vi "PH_PILS.panel.vi"(0 "object ref":refnum<vi>, 5 "error in (no error)":errorcluster) -> (19 "error out":errorcluster)   [LabVIEW 2014, in "PH_PILS.lvlib"]
doc: "By this VI a hardware switch can be monitored and switched. \n\nThe indicators \"FALSE\", \"TRUE\" and \"SWITCH STATE\" show the value of the Beckhoff-Tag: blue indicates bad tag status reference problems, darkgreen false and lightgreen true. If everything is working fine, \"FALSE\" and \"SWITCH STATE\" should show the same value, while \"TRUE\" has the opposite value. The caption of the sensors for \"FALSE\" and \"TRUE\" are taken out of the database. In case of only one or no sensor these GUI elements are not shown at all.\n\nThe oval button switches. It should be in the same state as the \"SWITCH STATE\" indicator. \n\n\"Delete Instance\" disconnects and removes the instance from the PCS.\n\n\nLicense Agreement for this software:\n\nCopyright (C)\nGesellschaft für Schwerionenforschung, GSI\nPlanckstr. 1\n64291 Darmstadt\nGermany\n\nContact: D.Beck@gsi.de \n\nThis program is free software; you can redistribute it and/or modify it under the terms of the GNU General Public License as published by the Free Software Foundation; either version 2 of the license, or (at your option) any later version.\n\nThis program is distributed in the hope that it will be useful, but WITHOUT ANYW ARRANTY; without even the implied warranty of MERCHANTABILITY or FITNESS FOR A PARTICULAR PURPOSE. See the GNU General License for more details (http://www.gnu.org).\n\nGesellschaft für Schwerionenforschung, GSI\nPlanckstr. 1, 64291 Darmstadt, Germany\nFor all questions and ideas contact: M.Richter@gsi.de, H.Brand@gsi.de or D.Beck@gsi.de.\nLast update: 18-DEC-2002"
uses:
  PH_PILS.lvlib
  PH_PILS.Submode.ctl
  PH_PILS.Operation Mode.ctl
  PH_Basics/PH_SystemInformation/PH_SystemInformation.GUI Refs.ctl
  PH_Basics/PH_Common/PH_Common.lvlib
  PH_Basics/PH_SystemInformation/PH_SystemInformation.lvlib
  PH_Basics/PH_Class/PH_Class.lvlib
  PH_Devices/PH_Beckhoff/PH_Beckhoff.lvlib
panel:
  out "PP_PA-19mm-2_DumpRoss_DE_closed_Slider":dbl(slide) scale=0.0..1.0
  out "PP_PA-19mm-1_DumpRoss_DE_closed_Slider":dbl(slide) scale=0.0..1.0
  out "PP_PA-19mm-2_DumpRoss_DE_closed":u32(colorbox)
  out "PP_PA-19mm-1_DumpRoss_DE_closed":u32(colorbox)
  out "PP_PA-19mm-2_PSU_DE_HV-on-indicator":u32(colorbox)
  out "PP_PA-19mm-1_PSU_DE_HV-on-indicator":u32(colorbox)
  out "PIL_NA_BeamdiagHVroom 2":bool caption="NA 6"
  out "PPPA_45mm_MAIN_DumpRoss_closed_Slider":dbl(slide) scale=0.0..1.0
  out "PPPA_45mm_PILC_DumpRoss_closed_Slider":dbl(slide) scale=0.0..1.0
  out "PP_PA-45mm-MAIN_DumpRoss_DE_closed":u32(colorbox)
  out "PP_PA-45mm-MAIN_PSU_DE_HV-on-indicator":u32(colorbox)
  out "PIL_DC_okPreamp":u32(colorbox)
  out "PP_Control_DC_ok":u32(colorbox)
  out "PA-19mm-Beckhoff-PU_DC_ok":u32(colorbox)
  out "PA-45mm-Beckhoff-PU_DC_ok":u32(colorbox)
  out "PIL_isOpen_T2_11":u32(colorbox)
  out "PIL_isOpen_T2_10":u32(colorbox)
  out "PIL_isOpen_T2_13":u32(colorbox)
  in  "PILo_unlock_HVDoor":bool caption="Unlock"
  in  "PILo_lock_HVDoor":bool caption="Lock"
  out "PIL_NA_BeamdiagHVroom 3":bool
  out "Mercury":u32(colorbox)=6618880 caption="23.99. 2013 08:55"
  out "PIL_Laserlab_bridged":bool caption="B"
  out "PIL_Laserbay_bridged":bool caption="B"
  in  "PILo_activate_laser_power":bool caption="Laser Suppy"
  out "PIL_Exp4_LaserEnabled":bool
  out "PIL_Exp3_LaserEnabled":bool
  out "PIL_Exp2_LaserEnabled":bool
  out "PIL_Exp1_LaserEnabled":bool
  in  "PILo_enable_AllLaser":bool
  out "PIL_disabled_laser":u32(colorbox)=16711680
  out "PPMA_Rods_b_down":u32(colorbox)
  out "PP_PA-45mm-PILC_DumpRoss_DE_closed":u32(colorbox)
  out "PIL_Shutter_Laserbay_closed":u32(colorbox)
  out "PIL_Shutter_Laserlab_closed":u32(colorbox)
  in  "PILo_activate_extEmergencies":bool
  out "PIL_Exp3_DoorOpen":u32(colorbox)
  out "PIL_Exp2_DoorOpen":u32(colorbox)
  out "PIL_Exp1_DoorOpen":u32(colorbox)
  out "MA01_O2_Lab_South_PreAlert":bool
  out "MA01_O2_Lab_North_PreAlert":bool
  out "MA-Rack4-Beckhoff-PU_DC_ok":u32(colorbox)
  out "PPMA_Rack5_DC_ok":u32(colorbox)
  out "PPMA_Rack4_DC_ok":u32(colorbox)
  out "PIL_NA_LaserLab 3":bool
  out "PA_Beckhoff-16BB_Flowbox_PA_on":bool
  out "PA_Beckhoff-16BB_Flowbox_fs_on":bool
  out "MA-Rack3-Beckhoff-PU_DC_ok":u32(colorbox)
  out "MA-Rack2-Beckhoff-PU_DC_ok":u32(colorbox)
  out "MA-Rack1-Beckhoff-PU_DC_ok":u32(colorbox)
  out "PILS_DE_earth-ok":u32(colorbox)
  out "PP_Rods_DE_watervalve-closed":bool
  out "Beamline Einschuss":u32(colorbox)
  out "PPPA_19mm_1_PSU_HV_on Head":u32(colorbox)
  out "PPPA_45mm_PSU_HV_on Head":u32(colorbox)
  out "PPPA_19mm_2_PSU_HV_on Head":u32(colorbox)
  out "PIL_shutter_fibre_closed":u32(colorbox)
  out "PIL_laserIL_deactiv 6":u32(colorbox)
  out "PIL_Lasergroup5_on 1":u32(colorbox)
  out "PIL_shutter_ns_closed":u32(colorbox)
  out "PIL_laserIL_deactiv 5":u32(colorbox)
  out "PIL_Lasergroup4_on":u32(colorbox)
  out "PIL_Lasergroup5_on 2":u32(colorbox)
  out "PIL_shutter_YLF_closed":u32(colorbox)
  out "PIL_laserIL_deactiv 4":u32(colorbox)
  out "PIL_Lasergroup2_on":u32(colorbox)
  out "PIL_shutter_Verdi_closed":u32(colorbox)
  out "PIL_laserIL_deactiv 3":u32(colorbox)
  out "PIL_Lasergroup3_on":u32(colorbox)
  out "PIL_shutter_8000B_closed":u32(colorbox)
  out "PIL_shutter_8000A_closed":u32(colorbox)
  out "PIL_laserIL_deactiv 2":u32(colorbox)
  out "PIL_shutter_9000B_closed":u32(colorbox)
  out "PIL_shutter_9000A_closed":u32(colorbox)
  out "PIL_laserIL_deactiv 1":u32(colorbox)
  out "PIL_Lasergroup1_on":u32(colorbox)
  out "Beamline Exp. 1":u32(colorbox)
  out "Beamline Exp. 2":u32(colorbox)
  out "Beamline Einschuss Exp. 1":u32(colorbox)
  out "Beamline Einschuss Exp. 2":u32(colorbox)
  out "Beamline Einschuss Exp. 3":u32(colorbox)
  out "Beamline Einschuss Exp. 4":u32(colorbox)
  out "Beamline Exp. 3":u32(colorbox)
  out "Beamline Exp. 4":u32(colorbox)
  out "Beamline Tower up":u32(colorbox)
  out "Beamline Bypass Booster":u32(colorbox)
  out "Beamline Tower/Exp":u32(colorbox)
  out "Beamline Faraday Rotator":u32(colorbox)=16711680
  out "Beamline Booster":u32(colorbox)
  out "Beamline Laserlab":u32(colorbox)
  out "Beamline MSF A":u32(colorbox)
  out "Beamline Turn MainAmp":u32(colorbox)
  out "Beamline MainAmp":u32(colorbox)
  out "PPMA_FR_PSU_HV_on Head":u32(colorbox)
  out "PPMA_PU6_PSU_HV_on Head":u32(colorbox)
  out "PPMA_PU7_PSU_HV_on Head":u32(colorbox)
  out "PPMA_PU8_PSU_HV_on Head":u32(colorbox)
  out "PPMA_PU9_PSU_HV_on Head":u32(colorbox)
  out "PPMA_PU10_PSU_HV_on Head":u32(colorbox)
  out "PPMA_PU5_PSU_HV_on Head":u32(colorbox)
  out "PPMA_PU4_PSU_HV_on Head":u32(colorbox)
  out "PPMA_PU3_PSU_HV_on Head":u32(colorbox)
  out "PPMA_PU2_PSU_HV_on Head":u32(colorbox)
  out "PPMA_PU1_PSU_HV_on Head":u32(colorbox)
  out "PPMA_Rods_a_down_Slider":dbl(slide) caption="Rods A" scale=0.0..1.0
  out "PPMA_Rods_b_down_Slider":dbl(slide) caption="Rods B" scale=0.0..1.0
  out "PPMA_Rods_a_down":u32(colorbox)
  out "PP_MA-PILC_PSU_DE_HV-on-indicator":u32(colorbox)=16860
  out "PP_MA-FR_PSU_DE_HV-on-indicator":u32(colorbox)=16860
  out "PPMA_PU10_PSU_HV_on":u32(colorbox)
  out "PPMA_PU9_PSU_HV_on":u32(colorbox)
  out "PPMA_PU8_PSU_HV_on":u32(colorbox)
  out "PPMA_PU7_PSU_HV_on":u32(colorbox)
  out "PP_MA-PU-6_PSU_DE_HV-on-indicator":u32(colorbox)
  out "PP_MA-PU-5_PSU_DE_HV-on-indicator":u32(colorbox)
  out "PP_MA-PU-4_PSU_DE_HV-on-indicator":u32(colorbox)
  out "PP_MA-PU-3_PSU_DE_HV-on-indicator":u32(colorbox)
  out "PP_MA-PU-2_PSU_DE_HV-on-indicator":u32(colorbox)
  out "PP_MA-PU-1_PSU_DE_HV-on-indicator":u32(colorbox)
  out "PILS_DE_door-locked-K2":u32(colorbox)
  out "PILS_DE_door-locked-K1":u32(colorbox)
  out "PIL_HVroom_locked":u32(colorbox)=16860
  in  "PILo_enable_exp4":bool
  out "PIL_Exp4_ShutterDisabled":u32(colorbox)
  in  "PILo_enable_exp3":bool
  out "PIL_Exp3_ShutterDisabled":u32(colorbox)
  in  "PILo_enable_exp2":bool
  out "PIL_Exp2_ShutterDisabled":u32(colorbox)
  in  "PILo_enable_exp1":bool
  out "PIL_Exp1_ShutterDisabled":u32(colorbox)
  in  "PILo_activate_MainEmergency":bool
  in  "PILo_enable_MainEmergency":bool=TRUE caption="Emergency Off"
  out "PIL_NA_Chain":u32(colorbox)
  in  "PILo_enable_Preamp":bool
  out "PIL_disabled_preamp":u32(colorbox)
  out "PIL_laserroom_ok":u32(colorbox) caption="Ack Laser Bay"
  out "PIL_HVroom_ok":u32(colorbox) caption="Ack HV"
  out "Exp":T1(ring)
  out "State Exp":u32(colorbox)
  out "Submode":T2
  out "State Submode":u32(colorbox)
  out "Operation Mode":T3
  out "State Operation Mode":u32(colorbox)
  out "PIL_Exp4_ShutterNotOpen":bool caption="Shutter not open"
  out "PIL_nhelix_on":bool caption="nhelix on"
  out "PIL_Exp4_DoorOpen":u32(colorbox)
  out "Exp. Shutter 4":dbl(slide) scale=0.0..1.0
  out "PIL_NA_Exp4":bool
  out "PIL_Exp4_ShutterNotClosed":bool caption="Shutter not closed"
  out "PIL_Exp3_ShutterNotOpen":bool caption="Shutter not open"
  out "Exp. Shutter 3":dbl(slide) scale=0.0..1.0
  out "PIL_NA_Exp3":bool
  out "PIL_Exp3_ShutterNotClosed":bool caption="Shutter not closed"
  out "PIL_Exp2_ShutterNotOpen":bool caption="Shutter not open"
  out "Exp. Shutter 2":dbl(slide) scale=0.0..1.0
  out "PIL_NA_Exp2":bool
  out "PIL_Exp2_ShutterNotClosed":bool caption="Shutter not closed"
  out "PIL_Exp1_ShutterNotOpen":bool caption="Shutter not open"
  out "Exp. Shutter 1":dbl(slide) scale=0.0..1.0
  out "PIL_NA_Exp1":bool
  out "PIL_Exp1_ShutterNotClosed":bool caption="Shutter not closed"
  out "PIL_PreAmp_keyswitch_1_002_on":u32(colorbox) caption="PP\nPA"
  out "PIL_MainAmp_keyswitch_1_002_on":u32(colorbox) caption="PP\nMA"
  out "PIL_MainAmp_keyswitch_2_005_on":u32(colorbox) caption="PP MA"
  out "PIL_DC_okA102":u32(colorbox)
  out "PPMA_Beckhoff-Dumprods_DC_ok":u32(colorbox)
  out "PIL_DC_ok11":u32(colorbox)
  out "PIL_DC_ok10":u32(colorbox)
  out "PIL_DC_ok9":u32(colorbox)
  out "PIL_DC_ok8":u32(colorbox)
  out "PIL_DC_ok7":u32(colorbox)
  out "PIL_DC_ok6":u32(colorbox)
  out "PIL_DC_ok5":u32(colorbox)
  out "PIL_DC_ok4":u32(colorbox)
  out "PIL_DC_ok3":u32(colorbox)
  out "PIL_DC_ok2":u32(colorbox)
  out "PIL_DC_ok1":u32(colorbox)
  out "PIL_NA_BeamdiagHVroom 5":bool
  out "PIL_NA_BeamdiagHVroom 4":bool
  out "PIL_enable_HVroom":bool
  in  "PILo_enable_mainamp":bool
  out "PIL_disabled_mainamp":u32(colorbox)
  out "PIL_enable_ELTroom":bool
  out "PIL_NA_LaserLab 2":bool
  out "PIL_NA_LaserLab 1":bool
  out "PIL_status_cerpass":u32(colorbox)
  out "PIL_isOpen_T1_09":u32(colorbox)
  out "PIL_isOpen_T1_10":u32(colorbox)
  out "PIL_isOpen_T1_04":u32(colorbox)
  out "PIL_isOpen_T1_05":u32(colorbox)
  out "PIL_isOpen_rollo":u32(colorbox)
  out "PIL_isOpen_T1_08":u32(colorbox)
  out "PIL_isOpen_T2_08":u32(colorbox)
  out "PIL_isOpen_T2_07":u32(colorbox)
  out "PIL_NA_PKR 1":bool
  out "PIL_NA_BeamdiagHVroom 6":bool
  out "PIL_NA_PKR 3":bool
  out "PIL_NA_PKR 2":bool
  out "PIL_NA_BeamdiagHVroom 1":bool
  out "PIL_NA_laserroom 4":bool
  out "PIL_NA_laserroom 3":bool
  out "PIL_NA_laserroom 2":bool
  out "PIL_NA_laserroom 1":bool
  out "PIL_enable_beamdiag":bool
  out "PIL_enable_laserlab":bool
  out "PIL_enable_laserroom 2":bool
  out "PIL_enable_laserroom 1":bool
  out "PIL_Exp1_MainampEnabled":bool
  out "PIL_Exp2_MainampEnabled":bool
  out "PIL_Exp3_MainampEnabled":bool
  out "PIL_Exp4_MainampEnabled":bool
  in  "Delete":bool
  # "PCS"
  # "3.40"
  # "Exp. 4 (Z6)"
  # "Experiment 1"
  # "Experiment 2"
  # "Experiment 3"
  # "LASER"
  # "Beam Diag.\nPLH 2.002"
  # "ELT  PLH 2.004"
  # "Laser Labor\nPLH 1.001"
  # "Test Labor\nPLH 2.001"
  # "HV"
  # "Stairway"
  # "Stairway"
  # "Laser Bay\nPLH 1.002"
  # "PKR\nPLH 2.007"
  # "PKR\nPLH 2.007a"
  # "HV Room\nPLH 2.005"
  # "Exp. 4 (Z6)"
  # "Exp. 3"
  # "Exp. 2"
  # "Exp. 1"
  # "EMERGENCY"
  # "PREAMP"
  # "MAINAMP"
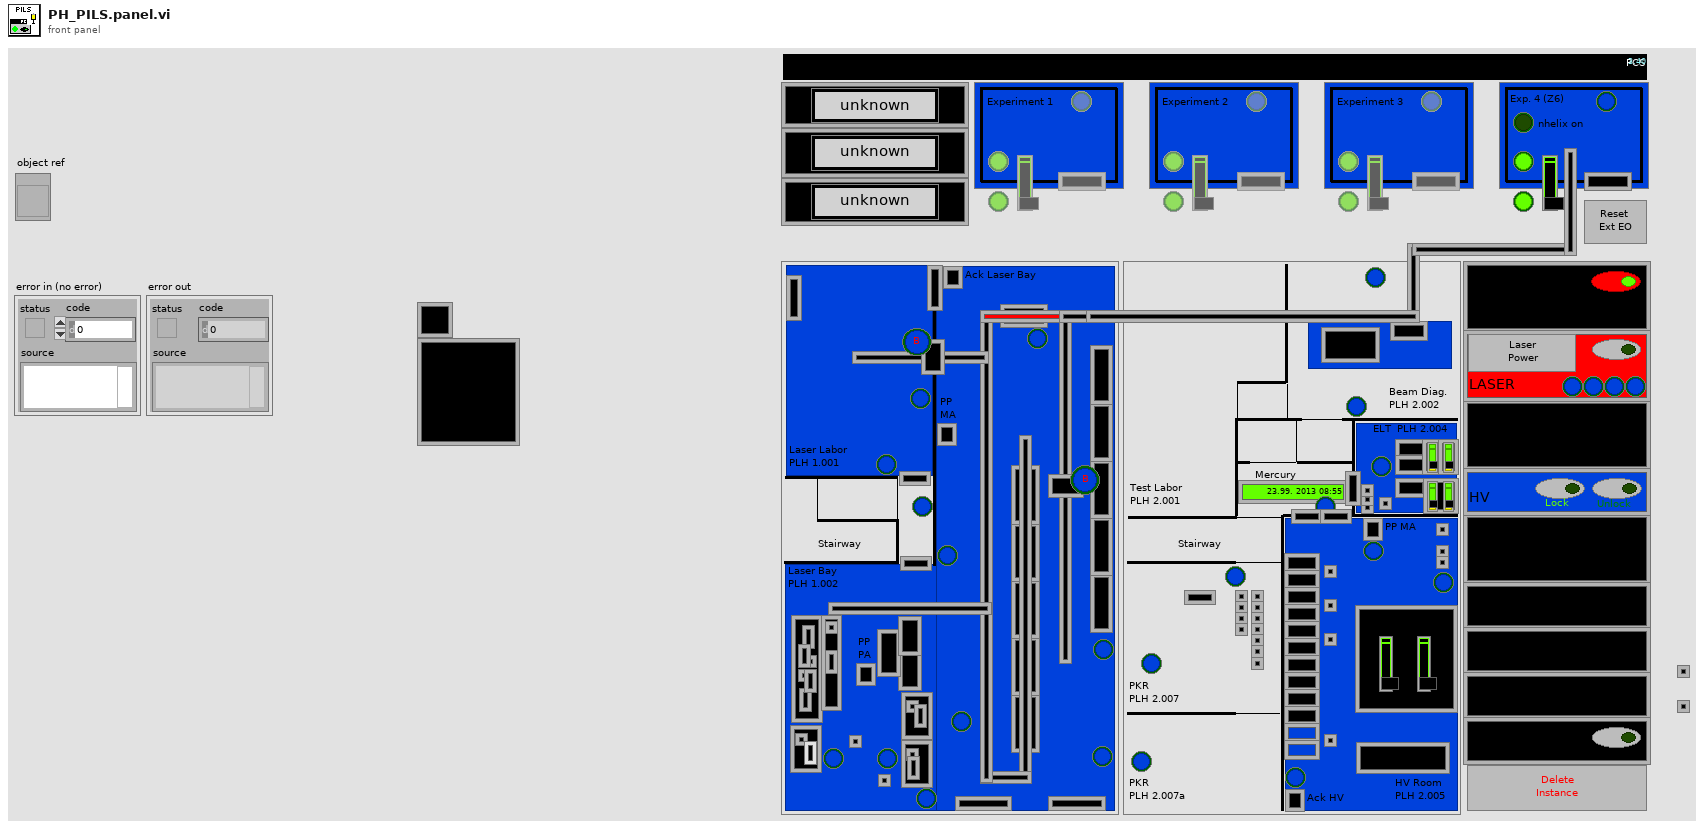
[diagram p1: front panel]
types:
  T1 = enum16{"unknown", "intern", "4 (Z6)", "3", "2", "1"}
  T2 = typedef "PH_PILS.lvlib/PH_PILS.Submode.ctl" = enum16{"unknown", "HV-Normal", "HV-Test"}
  T3 = typedef "PH_PILS.lvlib/PH_PILS.Operation Mode.ctl" = enum16{"unknown", "Service", "Labor", "Search", "Shot"}
  T4 = typedef "PH_SystemInformation.lvlib/PH_SystemInformation.GUI Refs.ctl" = cluster{"Laser":refnum<vi>, "PreAmp":refnum<vi>, "MainAmp":refnum<vi>, "Emergency Off":refnum<vi>, "Exp 1":refnum<vi>, "Exp 2":refnum<vi>, "Exp 3":refnum<vi>, "Exp 4":refnum<vi>, "Timing Mode GUI Ref":refnum<vi>}
  T5 = cluster{"GUI Ref":refnum<vi>, "Status":i32, "Head Ref":refnum<vi>, "Slider Ref":refnum<vi>}
  T6 = typedef "PH_PILS.lvlib/PH_PILS.i attribute.ctl" = cluster{"Boolean":cluster{"GUI Ref":refnum<vi>, "Status":i32}[], "GUI Refs Exp. Shutters":cluster{"1":refnum<vi>, "2":refnum<vi>, "3":refnum<vi>, "4":refnum<vi>}, "Tristate2Run GUI Refs":refnum<vi>[], "EO-Likes":cluster{"GUI Ref":refnum<vi>, "Status":i32}[], "Operation Mode":cluster{"Operation Mode":T3, "GUI":cluster{"Ref State":refnum<vi>, "Ref":refnum<vi>}, "Servicemode":cluster{"Tagname":string, "Status":i32}, "Labormode":cluster{"Tagname":string, "Status":i32}, "Searchmode":cluster{"Tagname":string, "Status":i32}, "Shotmode":cluster{"Tagname":string, "Status":i32}}, "Submode":cluster{"Submode":T2, "GUI":cluster{"Ref State":refnum<vi>, "Ref":refnum<vi>}, "Submode":cluster{"Tagname":string, "Status":i32}}, "Experiment":cluster{"Experiment":enum16{"unknown", "intern", "4 (Z6)", "3", "2", "1"}, "GUI":cluster{"Ref State":refnum<vi>, "Ref":refnum<vi>}, "intern":cluster{"Tagname":string, "Status":i32}, "Exp 4":cluster{"Tagname":string, "Status":i32}, "Exp 3":cluster{"Tagname":string, "Status":i32}, "Exp 2":cluster{"Tagname":string, "Status":i32}, "Exp 1":cluster{"Tagname":string, "Status":i32}}, "TristateNormal":cluster{"GUI Ref":refnum<vi>, "Status":i32}[], "Door Tags":cluster{"GUI Ref":refnum<vi>, "Status":i32}[], "GUIlessTags":cluster{"Name":string, "Status":i32}[], "Beamline GUI Refs":refnum<vi>[], "Special Boolean":cluster{"GUI Ref":refnum<vi>, "Status":i32}[], "Laserpower":cluster{"GUI Ref":refnum<vi>, "Status":i32}[], "Shutter":cluster{"GUI Ref":refnum<vi>, "Status":i32}[], "Tristate EO Like":cluster{"GUI Ref":refnum<vi>, "Status":i32}[], "PP":cluster{"GUI Ref":refnum<vi>, "Status":i32, "Head Ref":refnum<vi>, "Slider Ref":refnum<vi>}[], "Switch Knobs":cluster{"GUI Ref":refnum<vi>, "Status":i32}[], "Latch Knob GUI Refs":refnum<vi>[], "FailureCounter":i32, "Enabled Status":cluster{"Laser":i32, "PreAmp":i32, "MainAmp":i32}, "Mercury":refnum<vi>, "Instance Rods":string, "Logfile":path, "Beckhoff-Instance Internal":string, "Beckhoff-Instance External":string, "Enabling Rights":cluster{"Name":string, "Password":string, "PA?":bool, "MA?":bool, "Exp?":bool}[]}
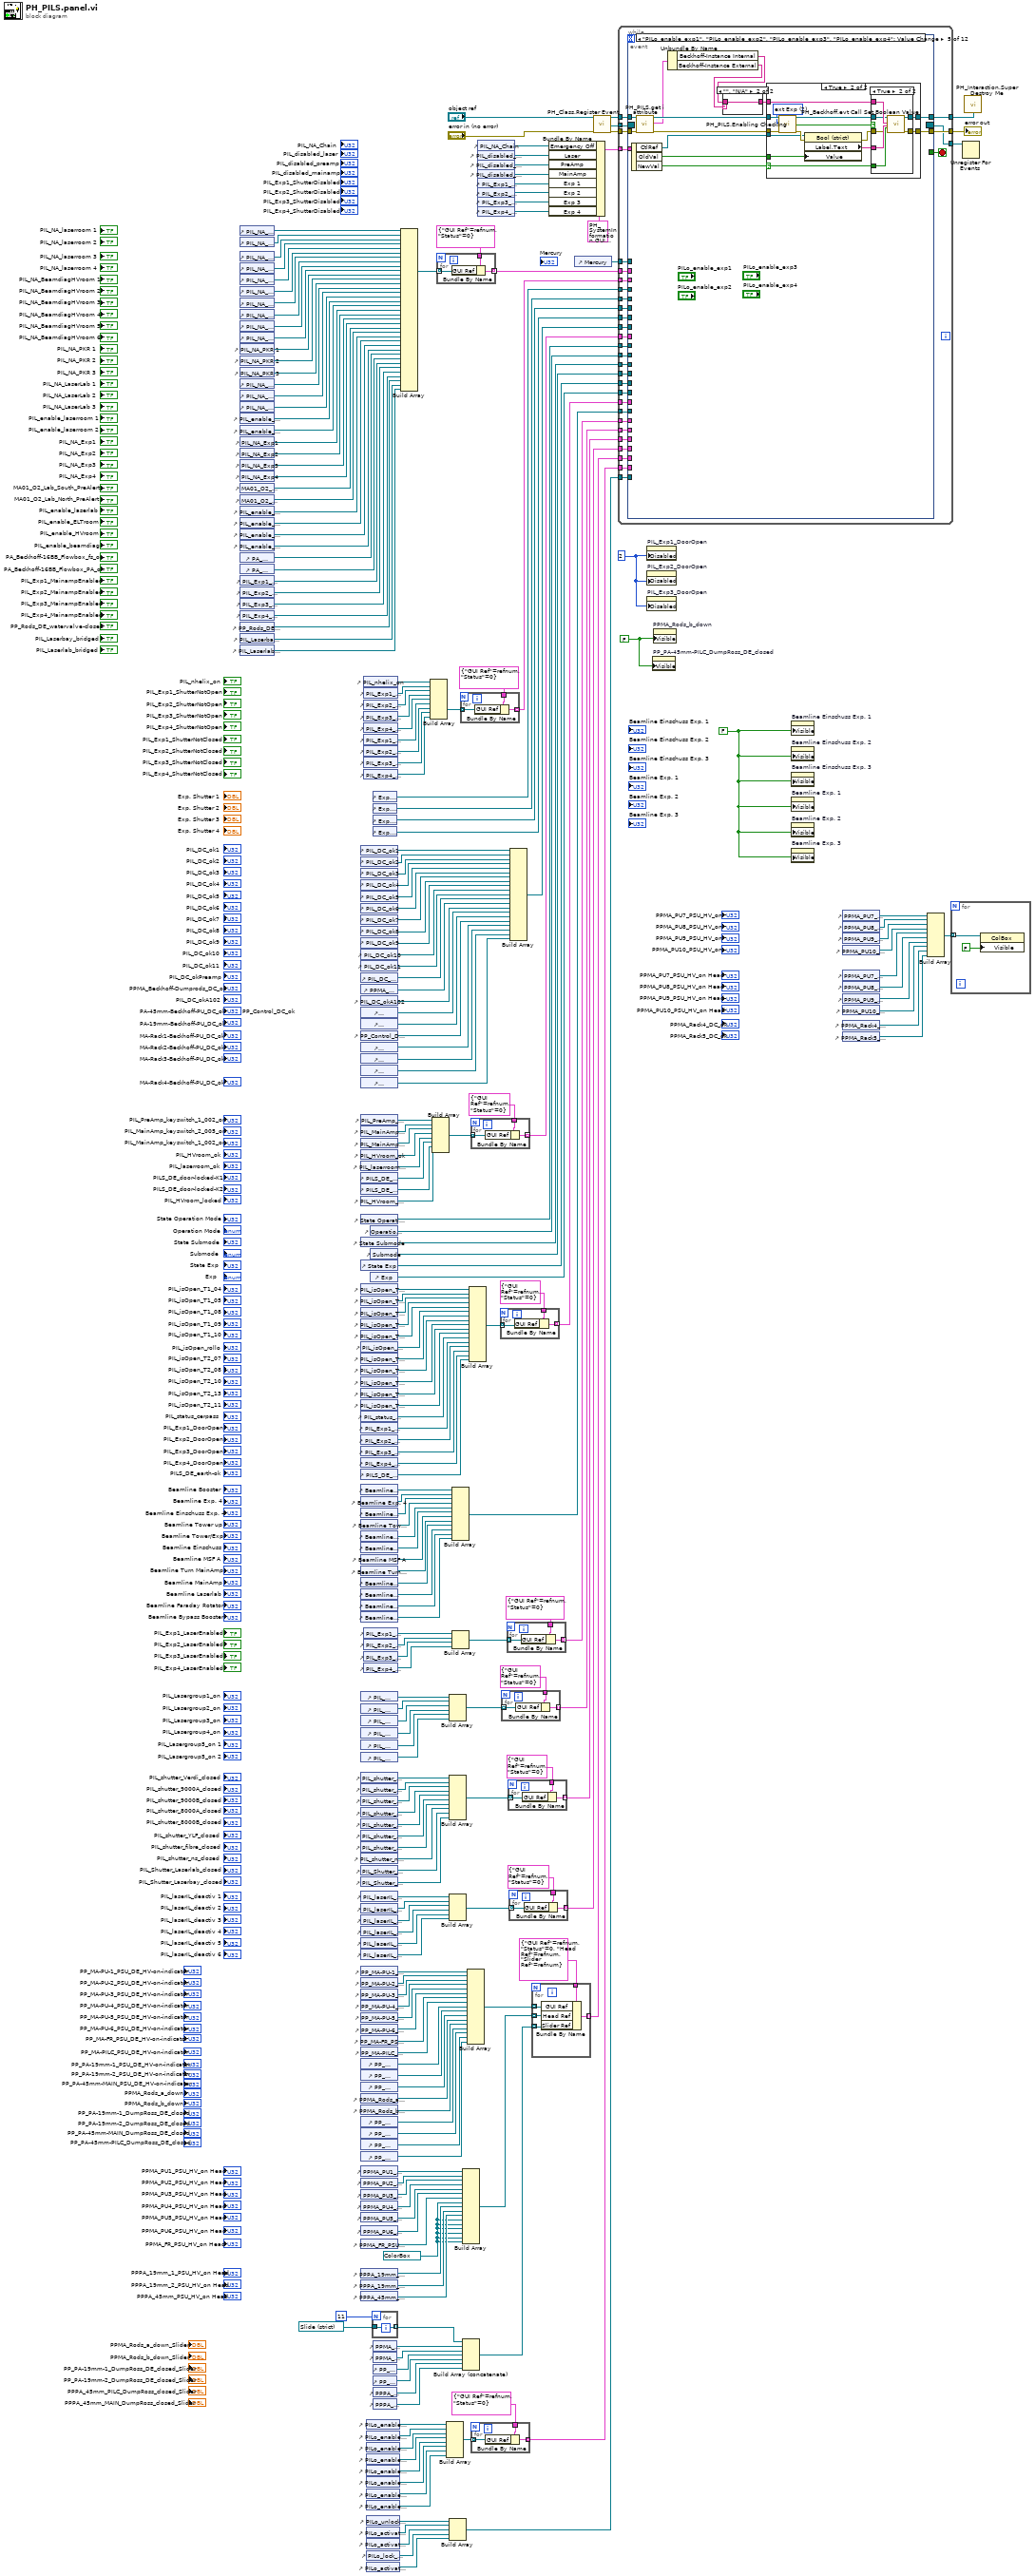
[diagram p0: block diagram]
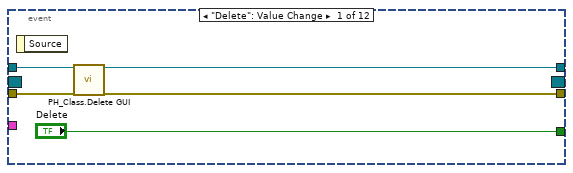
[diagram p2: hidden frame]
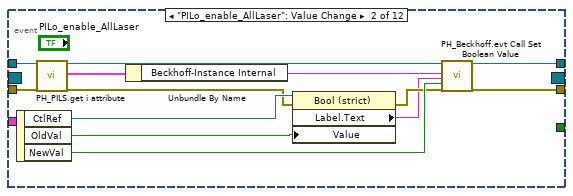
[diagram p3: hidden frame]
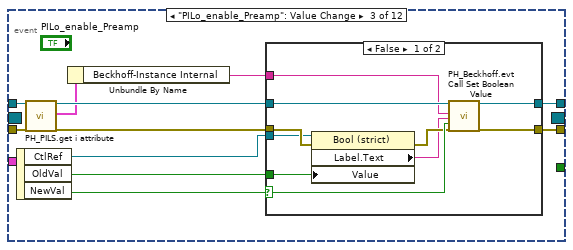
[diagram p4: hidden frame]
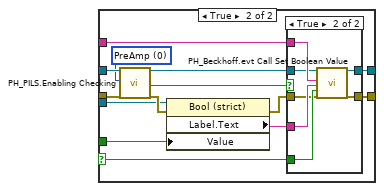
[diagram p5: hidden frame]
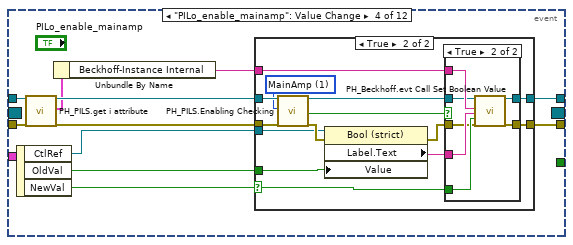
[diagram p7: hidden frame]
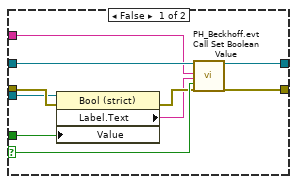
[diagram p8: hidden frame]
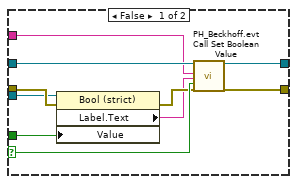
[diagram p11: hidden frame]
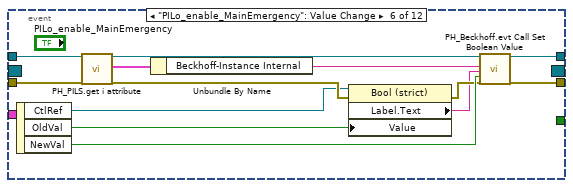
[diagram p13: hidden frame]
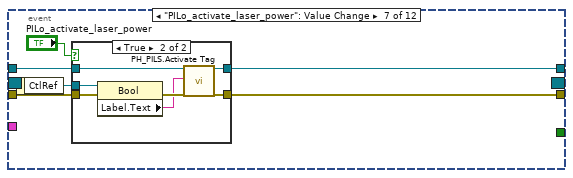
[diagram p14: hidden frame]
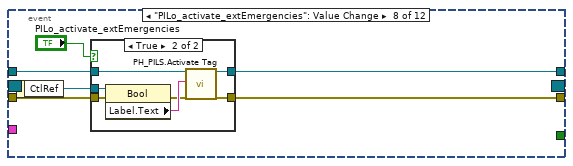
[diagram p16: hidden frame]
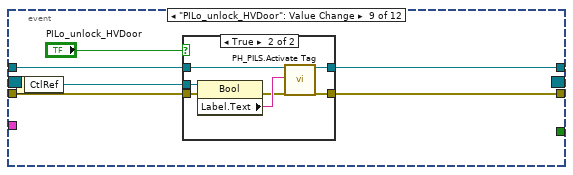
[diagram p18: hidden frame]
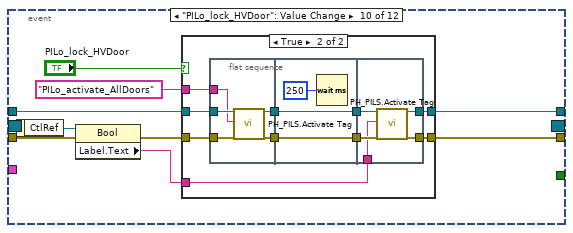
[diagram p20: hidden frame]
diagram:
  w77 = u8 2 ("Disabled")
  w90 = refnum<vi> refnum ("PPPA_45mm_PSU_HV_on Head")
  w98 = FALSE ("Visible")
  w171 = FALSE ("Visible")
  n1 = control-ref of="PIL_NA_laserroom 1"() -> (w257:refnum<vi>)
  n2 = control-ref of="PIL_NA_laserroom 2"() -> (w256:refnum<vi>)
  n3 = control-ref of="PIL_NA_laserroom 3"() -> (w255:refnum<vi>)
  n4 = control-ref of="PIL_NA_laserroom 4"() -> (w254:refnum<vi>)
  n5 = control-ref of="PIL_NA_BeamdiagHVroom 1"() -> (w253:refnum<vi>)
  n6 = control-ref of="PIL_NA_BeamdiagHVroom 2"() -> (w252:refnum<vi>)
  n7 = control-ref of="PIL_NA_BeamdiagHVroom 3"() -> (w251:refnum<vi>)
  n8 = control-ref of="PIL_NA_BeamdiagHVroom 4"() -> (w250:refnum<vi>)
  n9 = control-ref of="PIL_NA_BeamdiagHVroom 5"() -> (w249:refnum<vi>)
  n10 = control-ref of="PIL_NA_BeamdiagHVroom 6"() -> (w248:refnum<vi>)
  n11 = control-ref of="PIL_NA_PKR 1"() -> (w247:refnum<vi>)
  n12 = control-ref of="PIL_NA_PKR 2"() -> (w246:refnum<vi>)
  n13 = control-ref of="PIL_NA_PKR 3"() -> (w245:refnum<vi>)
  n14 = control-ref of="PIL_NA_LaserLab 1"() -> (w244:refnum<vi>)
  n15 = control-ref of="PIL_NA_LaserLab 2"() -> (w243:refnum<vi>)
  n16 = control-ref of="PIL_NA_LaserLab 3"() -> (w242:refnum<vi>)
  n17 = control-ref of="PIL_enable_laserroom 1"() -> (w241:refnum<vi>)
  n18 = control-ref of="PIL_enable_laserroom 2"() -> (w240:refnum<vi>)
  n19 = control-ref of="PIL_NA_Exp1"() -> (w239:refnum<vi>)
  n20 = control-ref of="PIL_NA_Exp2"() -> (w238:refnum<vi>)
  n21 = control-ref of="PIL_NA_Exp3"() -> (w237:refnum<vi>)
  n22 = control-ref of="PIL_NA_Exp4"() -> (w236:refnum<vi>)
  n23 = control-ref of="MA01_O2_Lab_South_PreAlert"() -> (w235:refnum<vi>)
  n24 = control-ref of="MA01_O2_Lab_North_PreAlert"() -> (w234:refnum<vi>)
  n25 = control-ref of="PIL_enable_laserlab"() -> (w233:refnum<vi>)
  n26 = control-ref of="PIL_enable_ELTroom"() -> (w232:refnum<vi>)
  n27 = control-ref of="PIL_enable_HVroom"() -> (w231:refnum<vi>)
  n28 = control-ref of="PIL_enable_beamdiag"() -> (w230:refnum<vi>)
  n29 = control-ref of="PA_Beckhoff-16BB_Flowbox_fs_on"() -> (w229:refnum<vi>)
  n30 = control-ref of="PA_Beckhoff-16BB_Flowbox_PA_on"() -> (w228:refnum<vi>)
  n31 = control-ref of="PIL_Exp1_MainampEnabled"() -> (w227:refnum<vi>)
  n32 = control-ref of="PIL_Exp2_MainampEnabled"() -> (w226:refnum<vi>)
  n33 = control-ref of="PIL_Exp3_MainampEnabled"() -> (w225:refnum<vi>)
  n34 = control-ref of="PIL_Exp4_MainampEnabled"() -> (w224:refnum<vi>)
  n35 = control-ref of="PP_Rods_DE_watervalve-closed"() -> (w223:refnum<vi>)
  n36 = control-ref of="PIL_Laserbay_bridged"() -> (w47:refnum<vi>)
  n37 = control-ref of="PIL_Laserlab_bridged"() -> (w46:refnum<vi>)
  n38 = control-ref of="PIL_DC_ok1"() -> (w211:refnum<vi>)
  n39 = control-ref of="PIL_DC_ok2"() -> (w210:refnum<vi>)
  n40 = control-ref of="PIL_DC_ok3"() -> (w209:refnum<vi>)
  n41 = control-ref of="PIL_DC_ok4"() -> (w208:refnum<vi>)
  n42 = control-ref of="PIL_DC_ok5"() -> (w207:refnum<vi>)
  n43 = control-ref of="PIL_DC_ok6"() -> (w206:refnum<vi>)
  n44 = control-ref of="PIL_DC_ok7"() -> (w205:refnum<vi>)
  n45 = control-ref of="PIL_DC_ok8"() -> (w204:refnum<vi>)
  n46 = control-ref of="PIL_DC_ok9"() -> (w203:refnum<vi>)
  n47 = control-ref of="PIL_DC_ok10"() -> (w202:refnum<vi>)
  n48 = control-ref of="PIL_DC_ok11"() -> (w201:refnum<vi>)
  n49 = control-ref of="PIL_DC_okPreamp"() -> (w200:refnum<vi>)
  n50 = control-ref of="PPMA_Beckhoff-Dumprods_DC_ok"() -> (w199:refnum<vi>)
  n51 = control-ref of="PIL_DC_okA102"() -> (w198:refnum<vi>)
  n52 = control-ref of="PA-45mm-Beckhoff-PU_DC_ok"() -> (w197:refnum<vi>)
  n53 = control-ref of="PA-19mm-Beckhoff-PU_DC_ok"() -> (w196:refnum<vi>)
  n54 = control-ref of="PP_Control_DC_ok"() -> (w195:refnum<vi>)
  n55 = control-ref of="MA-Rack1-Beckhoff-PU_DC_ok"() -> (w60:refnum<vi>)
  n56 = control-ref of="MA-Rack2-Beckhoff-PU_DC_ok"() -> (w59:refnum<vi>)
  n57 = control-ref of="MA-Rack3-Beckhoff-PU_DC_ok"() -> (w58:refnum<vi>)
  n58 = control-ref of="MA-Rack4-Beckhoff-PU_DC_ok"() -> (w57:refnum<vi>)
  n59 = control-ref of="PIL_PreAmp_keyswitch_1_002_on"() -> (w194:refnum<vi>)
  n60 = control-ref of="PIL_MainAmp_keyswitch_2_005_on"() -> (w193:refnum<vi>)
  n61 = control-ref of="PIL_MainAmp_keyswitch_1_002_on"() -> (w192:refnum<vi>)
  n62 = control-ref of="PIL_HVroom_ok"() -> (w191:refnum<vi>)
  n63 = control-ref of="PIL_laserroom_ok"() -> (w190:refnum<vi>)
  n64 = control-ref of="PILS_DE_door-locked-K1"() -> (w189:refnum<vi>)
  n65 = control-ref of="PILS_DE_door-locked-K2"() -> (w188:refnum<vi>)
  n66 = control-ref of="PIL_HVroom_locked"() -> (w130:refnum<vi>)
  n67 = control-ref of="State Operation Mode"() -> (w15:refnum<vi>)
  n68 = control-ref of="State Submode"() -> (w13:refnum<vi>)
  n69 = control-ref of="State Exp"() -> (w11:refnum<vi>)
  n70 = control-ref of="PIL_isOpen_T1_04"() -> (w183:refnum<vi>)
  n71 = control-ref of="PIL_isOpen_T1_05"() -> (w182:refnum<vi>)
  n72 = control-ref of="PIL_isOpen_T1_08"() -> (w181:refnum<vi>)
  n73 = control-ref of="PIL_isOpen_T1_09"() -> (w180:refnum<vi>)
  n74 = control-ref of="PIL_isOpen_T1_10"() -> (w144:refnum<vi>)
  n75 = control-ref of="PIL_isOpen_rollo"() -> (w179:refnum<vi>)
  n76 = control-ref of="PIL_isOpen_T2_07"() -> (w178:refnum<vi>)
  n77 = control-ref of="PIL_isOpen_T2_08"() -> (w177:refnum<vi>)
  n78 = control-ref of="PIL_isOpen_T2_10"() -> (w176:refnum<vi>)
  n79 = control-ref of="PIL_isOpen_T2_13"() -> (w175:refnum<vi>)
  n80 = control-ref of="PIL_isOpen_T2_11"() -> (w174:refnum<vi>)
  n81 = control-ref of="PIL_status_cerpass"() -> (w173:refnum<vi>)
  n82 = control-ref of="PIL_Exp1_DoorOpen"() -> (w121:refnum<vi>)
  n83 = control-ref of="PIL_Exp2_DoorOpen"() -> (w120:refnum<vi>)
  n84 = control-ref of="PIL_Exp3_DoorOpen"() -> (w119:refnum<vi>)
  n85 = control-ref of="PIL_Exp4_DoorOpen"() -> (w118:refnum<vi>)
  n86 = control-ref of="PILS_DE_earth-ok"() -> (w78:refnum<vi>)
  n87 = control-ref of="Beamline Booster"() -> (w170:refnum<vi>)
  n88 = control-ref of="Beamline Exp. 4"() -> (w169:refnum<vi>)
  n89 = control-ref of="Beamline Einschuss Exp. 4"() -> (w168:refnum<vi>)
  n90 = control-ref of="Beamline Tower up"() -> (w167:refnum<vi>)
  n91 = control-ref of="Beamline Tower/Exp"() -> (w166:refnum<vi>)
  n92 = control-ref of="Beamline Einschuss"() -> (w165:refnum<vi>)
  n93 = control-ref of="Beamline MSF A"() -> (w164:refnum<vi>)
  n94 = control-ref of="Beamline Turn MainAmp"() -> (w163:refnum<vi>)
  n95 = control-ref of="Beamline MainAmp"() -> (w162:refnum<vi>)
  n96 = control-ref of="Beamline Laserlab"() -> (w161:refnum<vi>)
  n97 = control-ref of="Beamline Faraday Rotator"() -> (w160:refnum<vi>)
  n98 = control-ref of="Beamline Bypass Booster"() -> (w159:refnum<vi>)
  n99 = control-ref of="PIL_Lasergroup1_on"() -> (w152:refnum<vi>)
  n100 = control-ref of="PIL_Lasergroup2_on"() -> (w151:refnum<vi>)
  n101 = control-ref of="PIL_Lasergroup3_on"() -> (w150:refnum<vi>)
  n102 = control-ref of="PIL_Lasergroup4_on"() -> (w149:refnum<vi>)
  n103 = control-ref of="PIL_Lasergroup5_on 1"() -> (w148:refnum<vi>)
  n104 = control-ref of="PIL_Lasergroup5_on 2"() -> (w147:refnum<vi>)
  n105 = control-ref of="PIL_shutter_Verdi_closed"() -> (w143:refnum<vi>)
  n106 = control-ref of="PIL_shutter_9000A_closed"() -> (w142:refnum<vi>)
  n107 = control-ref of="PIL_shutter_9000B_closed"() -> (w141:refnum<vi>)
  n108 = control-ref of="PIL_shutter_8000A_closed"() -> (w140:refnum<vi>)
  n109 = control-ref of="PIL_shutter_8000B_closed"() -> (w139:refnum<vi>)
  n110 = control-ref of="PIL_shutter_YLF_closed"() -> (w138:refnum<vi>)
  n111 = control-ref of="PIL_shutter_fibre_closed"() -> (w137:refnum<vi>)
  n112 = control-ref of="PIL_shutter_ns_closed"() -> (w136:refnum<vi>)
  n113 = control-ref of="PIL_Shutter_Laserlab_closed"() -> (w135:refnum<vi>)
  n114 = control-ref of="PIL_Shutter_Laserbay_closed"() -> (w134:refnum<vi>)
  n115 = control-ref of="PIL_laserIL_deactiv 1"() -> (w129:refnum<vi>)
  n116 = control-ref of="PIL_laserIL_deactiv 2"() -> (w128:refnum<vi>)
  n117 = control-ref of="PIL_laserIL_deactiv 3"() -> (w127:refnum<vi>)
  n118 = control-ref of="PIL_laserIL_deactiv 4"() -> (w126:refnum<vi>)
  n119 = control-ref of="PIL_laserIL_deactiv 5"() -> (w124:refnum<vi>)
  n120 = control-ref of="PIL_laserIL_deactiv 6"() -> (w125:refnum<vi>)
  n121 = control-ref of="PP_MA-PU-1_PSU_DE_HV-on-indicator"() -> (w117:refnum<vi>)
  n122 = control-ref of="PP_MA-PU-2_PSU_DE_HV-on-indicator"() -> (w116:refnum<vi>)
  n123 = control-ref of="PP_MA-PU-3_PSU_DE_HV-on-indicator"() -> (w115:refnum<vi>)
  n124 = control-ref of="PP_MA-PU-4_PSU_DE_HV-on-indicator"() -> (w114:refnum<vi>)
  n125 = control-ref of="PP_MA-PU-5_PSU_DE_HV-on-indicator"() -> (w113:refnum<vi>)
  n126 = control-ref of="PP_MA-PU-6_PSU_DE_HV-on-indicator"() -> (w34:refnum<vi>)
  n127 = control-ref of="PP_MA-FR_PSU_DE_HV-on-indicator"() -> (w112:refnum<vi>)
  n128 = control-ref of="PP_MA-PILC_PSU_DE_HV-on-indicator"() -> (w33:refnum<vi>)
  n129 = control-ref of="PP_PA-19mm-1_PSU_DE_HV-on-indicator"() -> (w111:refnum<vi>)
  n130 = control-ref of="PP_PA-19mm-2_PSU_DE_HV-on-indicator"() -> (w110:refnum<vi>)
  n131 = control-ref of="PP_PA-45mm-MAIN_PSU_DE_HV-on-indicator"() -> (w109:refnum<vi>)
  n132 = control-ref of="PPMA_Rods_a_down"() -> (w97:refnum<vi>)
  n133 = control-ref of="PPMA_Rods_b_down"() -> (w96:refnum<vi>)
  n134 = control-ref of="PP_PA-19mm-1_DumpRoss_DE_closed"() -> (w95:refnum<vi>)
  n135 = control-ref of="PP_PA-19mm-2_DumpRoss_DE_closed"() -> (w94:refnum<vi>)
  n136 = control-ref of="PP_PA-45mm-MAIN_DumpRoss_DE_closed"() -> (w93:refnum<vi>)
  n137 = control-ref of="PP_PA-45mm-PILC_DumpRoss_DE_closed"() -> (w92:refnum<vi>)
  n138 = control-ref of="PPMA_PU1_PSU_HV_on Head"() -> (w107:refnum<vi>)
  n139 = control-ref of="PPMA_PU2_PSU_HV_on Head"() -> (w106:refnum<vi>)
  n140 = control-ref of="PPMA_PU3_PSU_HV_on Head"() -> (w105:refnum<vi>)
  n141 = control-ref of="PPMA_PU4_PSU_HV_on Head"() -> (w104:refnum<vi>)
  n142 = control-ref of="PPMA_PU5_PSU_HV_on Head"() -> (w103:refnum<vi>)
  n143 = control-ref of="PPMA_PU6_PSU_HV_on Head"() -> (w32:refnum<vi>)
  n144 = control-ref of="PPMA_FR_PSU_HV_on Head"() -> (w102:refnum<vi>)
  n145 = control-ref of="PPPA_19mm_1_PSU_HV_on Head"() -> (w101:refnum<vi>)
  n146 = control-ref of="PPPA_19mm_2_PSU_HV_on Head"() -> (w100:refnum<vi>)
  n147 = control-ref of="PPPA_45mm_PSU_HV_on Head"() -> (w99:refnum<vi>)
  n148 = control-ref of="PIL_nhelix_on"() -> (w222:refnum<vi>)
  n149 = control-ref of="PIL_Exp1_ShutterNotOpen"() -> (w221:refnum<vi>)
  n150 = control-ref of="PIL_Exp2_ShutterNotOpen"() -> (w220:refnum<vi>)
  n151 = control-ref of="PIL_Exp3_ShutterNotOpen"() -> (w219:refnum<vi>)
  n152 = control-ref of="PIL_Exp4_ShutterNotOpen"() -> (w218:refnum<vi>)
  n153 = control-ref of="PIL_Exp1_ShutterNotClosed"() -> (w217:refnum<vi>)
  n154 = control-ref of="PIL_Exp2_ShutterNotClosed"() -> (w216:refnum<vi>)
  n155 = control-ref of="PIL_Exp3_ShutterNotClosed"() -> (w215:refnum<vi>)
  n156 = control-ref of="PIL_Exp4_ShutterNotClosed"() -> (w214:refnum<vi>)
  n157 = control-ref of="PIL_Exp1_LaserEnabled"() -> (w158:refnum<vi>)
  n158 = control-ref of="PIL_Exp2_LaserEnabled"() -> (w157:refnum<vi>)
  n159 = control-ref of="PIL_Exp3_LaserEnabled"() -> (w156:refnum<vi>)
  n160 = control-ref of="PIL_Exp4_LaserEnabled"() -> (w155:refnum<vi>)
  n161 = control-ref of="PILo_enable_MainEmergency"() -> (w76:refnum<vi>)
  n162 = control-ref of="PILo_enable_AllLaser"() -> (w75:refnum<vi>)
  n163 = control-ref of="PILo_enable_Preamp"() -> (w74:refnum<vi>)
  n164 = control-ref of="PILo_enable_mainamp"() -> (w73:refnum<vi>)
  n165 = control-ref of="PILo_enable_exp1"() -> (w72:refnum<vi>)
  n166 = control-ref of="PILo_enable_exp2"() -> (w71:refnum<vi>)
  n167 = control-ref of="PILo_enable_exp3"() -> (w67:refnum<vi>)
  n168 = control-ref of="PILo_enable_exp4"() -> (w70:refnum<vi>)
  n169 = control-ref of="PILo_unlock_HVDoor"() -> (w66:refnum<vi>)
  n170 = control-ref of="PILo_activate_MainEmergency"() -> (w65:refnum<vi>)
  n171 = control-ref of="PILo_activate_extEmergencies"() -> (w64:refnum<vi>)
  n172 = control-ref of="PILo_lock_HVDoor"() -> (w63:refnum<vi>)
  n173 = control-ref of="PILo_activate_laser_power"() -> (w62:refnum<vi>)
  n174 = control-ref of="Operation Mode"() -> (w14:refnum<vi>)
  n175 = control-ref of="Submode"() -> (w12:refnum<vi>)
  n176 = control-ref of="Exp"() -> (w10:refnum<vi>)
  n177 = for {
    N: 11 -> [_]
    tunnel: [w259] -> w80 mode=indexing
    tunnel: refnum<vi> refnum ("PPPA_19mm_1_DumpRoss_closed_Slider") -> [w259]
  }
  n178 = control-ref of="Exp. Shutter 1"() -> (w21:refnum<vi>)
  n179 = control-ref of="Exp. Shutter 2"() -> (w20:refnum<vi>)
  n180 = control-ref of="Exp. Shutter 3"() -> (w19:refnum<vi>)
  n181 = control-ref of="Exp. Shutter 4"() -> (w18:refnum<vi>)
  n182 = control-ref of="PPMA_Rods_a_down_Slider"() -> (w84:refnum<vi>)
  n183 = control-ref of="PPMA_Rods_b_down_Slider"() -> (w83:refnum<vi>)
  n184 = control-ref of="PP_PA-19mm-1_DumpRoss_DE_closed_Slider"() -> (w89:refnum<vi>)
  n185 = control-ref of="PP_PA-19mm-2_DumpRoss_DE_closed_Slider"() -> (w88:refnum<vi>)
  n186 = control-ref of="PPPA_45mm_PILC_DumpRoss_closed_Slider"() -> (w87:refnum<vi>)
  n187 = control-ref of="PPPA_45mm_MAIN_DumpRoss_closed_Slider"() -> (w86:refnum<vi>)
  n188 = Build Array(w257, w256, w255, w254, w253, w252, w251, w250, w249, w248, w247, w246, w245, w244, w243, w242, w241, w240, w239, w238, w237, w236, w235, w234, w233, w232, w231, w230, w229, w228, w227, w226, w225, w224, w223, w47, w46) -> (w186:refnum<vi>[])
  n189 = Build Array(w222, w221, w220, w219, w218, w217, w216, w215, w214) -> (w213:refnum<vi>[])
  n190 = Build Array(w194, w193, w192, w191, w190, w189, w188, w130) -> (w185:refnum<vi>[])
  n191 = for {
    tunnel: cluster{"GUI Ref":refnum<vi>, "Status":i32} {"GUI Ref"=refnum, "Status"=0} ("Cluster") -> [w262]
    tunnel: w186 -> [w260] mode=indexing
    tunnel: [w261] -> w23 mode=indexing
    n192 = Bundle By Name(cluster=w262, "GUI Ref"=w260) -> (w261:cluster{"GUI Ref":refnum<vi>, "Status":i32})
  }
  n193 = Build Array(w76, w75, w74, w73, w72, w71, w67, w70) -> (w68:refnum<vi>[])
  n194 = Build Array(w66, w65, w64, w63, w62) -> (w1:refnum<vi>[])
  n195 = Build Array(w152, w151, w150, w149, w148, w147) -> (w145:refnum<vi>[])
  n196 = Build Array(w143, w142, w141, w140, w139, w138, w137, w136, w135, w134) -> (w132:refnum<vi>[])
  n197 = Build Array(w129, w128, w127, w126, w124, w125) -> (w122:refnum<vi>[])
  n198 = Build Array(w170, w169, w168, w167, w166, w165, w164, w163, w162, w161, w160, w159) -> (w8:refnum<vi>[])
  n199 = Build Array(w158, w157, w156, w155) -> (w153:refnum<vi>[])
  n200 = for {
    tunnel: cluster{"GUI Ref":refnum<vi>, "Status":i32} {"GUI Ref"=refnum, "Status"=0} ("Cluster") -> [w265]
    tunnel: w213 -> [w263] mode=indexing
    tunnel: [w264] -> w22 mode=indexing
    n201 = Bundle By Name(cluster=w265, "GUI Ref"=w263) -> (w264:cluster{"GUI Ref":refnum<vi>, "Status":i32})
  }
  n202 = Build Array(w107, w106, w105, w104, w103, w32, w102, w90, w101, w100, w99, w90, w90, w90, w90, w90, w90) -> (w91:refnum<vi>[])
  n203 = Build Array (concatenate)(w80, w84, w83, w89, w88, w87, w86) -> (w79:refnum<vi>[])
  n204 = Build Array(w117, w116, w115, w114, w113, w34, w112, w33, w111, w110, w109, w97, w96, w95, w94, w93, w92) -> (w108:refnum<vi>[])
  n205 = Build Array(w183, w182, w181, w180, w144, w179, w178, w177, w176, w175, w174, w173, w121, w120, w119, w118, w78) -> (w172:refnum<vi>[])
  n206 = for {
    tunnel: cluster{"GUI Ref":refnum<vi>, "Status":i32} {"GUI Ref"=refnum, "Status"=0} ("element") -> [w268]
    tunnel: w185 -> [w266] mode=indexing
    tunnel: [w267] -> w16 mode=indexing
    n207 = Bundle By Name(cluster=w268, "GUI Ref"=w266) -> (w267:cluster{"GUI Ref":refnum<vi>, "Status":i32})
  }
  n208 = for {
    tunnel: cluster{"GUI Ref":refnum<vi>, "Status":i32} {"GUI Ref"=refnum, "Status"=0} ("Cluster") -> [w271]
    tunnel: [w270] -> w2 mode=indexing
    tunnel: w68 -> [w269] mode=indexing
    n209 = Bundle By Name(cluster=w271, "GUI Ref"=w269) -> (w270:cluster{"GUI Ref":refnum<vi>, "Status":i32})
  }
  n210 = control-ref of="PIL_NA_Chain"() -> (w55:refnum<vi>)
  n211 = control-ref of="PIL_disabled_laser"() -> (w54:refnum<vi>)
  n212 = control-ref of="PIL_disabled_preamp"() -> (w53:refnum<vi>)
  n213 = control-ref of="PIL_disabled_mainamp"() -> (w52:refnum<vi>)
  n214 = control-ref of="PIL_Exp1_ShutterDisabled"() -> (w51:refnum<vi>)
  n215 = control-ref of="PIL_Exp2_ShutterDisabled"() -> (w50:refnum<vi>)
  n216 = control-ref of="PIL_Exp3_ShutterDisabled"() -> (w49:refnum<vi>)
  n217 = control-ref of="PIL_Exp4_ShutterDisabled"() -> (w48:refnum<vi>)
  n218 = for {
    tunnel: cluster{"GUI Ref":refnum<vi>, "Status":i32} {"GUI Ref"=refnum, "Status"=0} ("element") -> [w274]
    tunnel: w172 -> [w272] mode=indexing
    tunnel: [w273] -> w9 mode=indexing
    n219 = Bundle By Name(cluster=w274, "GUI Ref"=w272) -> (w273:cluster{"GUI Ref":refnum<vi>, "Status":i32})
  }
  n220 = for {
    tunnel: cluster{"GUI Ref":refnum<vi>, "Status":i32} {"GUI Ref"=refnum, "Status"=0} ("element") -> [w277]
    tunnel: w145 -> [w275] mode=indexing
    tunnel: [w276] -> w6 mode=indexing
    n221 = Bundle By Name(cluster=w277, "GUI Ref"=w275) -> (w276:cluster{"GUI Ref":refnum<vi>, "Status":i32})
  }
  n222 = for {
    tunnel: cluster{"GUI Ref":refnum<vi>, "Status":i32} {"GUI Ref"=refnum, "Status"=0} ("Cluster") -> [w280]
    tunnel: w153 -> [w278] mode=indexing
    tunnel: [w279] -> w7 mode=indexing
    n223 = Bundle By Name(cluster=w280, "GUI Ref"=w278) -> (w279:cluster{"GUI Ref":refnum<vi>, "Status":i32})
  }
  n224 = for {
    tunnel: cluster{"GUI Ref":refnum<vi>, "Status":i32} {"GUI Ref"=refnum, "Status"=0} ("element") -> [w283]
    tunnel: w132 -> [w281] mode=indexing
    tunnel: [w282] -> w5 mode=indexing
    n225 = Bundle By Name(cluster=w283, "GUI Ref"=w281) -> (w282:cluster{"GUI Ref":refnum<vi>, "Status":i32})
  }
  n226 = for {
    tunnel: cluster{"GUI Ref":refnum<vi>, "Status":i32} {"GUI Ref"=refnum, "Status"=0} ("element") -> [w286]
    tunnel: w122 -> [w284] mode=indexing
    tunnel: [w285] -> w4 mode=indexing
    n227 = Bundle By Name(cluster=w286, "GUI Ref"=w284) -> (w285:cluster{"GUI Ref":refnum<vi>, "Status":i32})
  }
  n228 = Build Array(w211, w210, w209, w208, w207, w206, w205, w204, w203, w202, w201, w200, w199, w198, w197, w196, w195, w60, w59, w58, w57) -> (w17:refnum<vi>[])
  n229 = for {
    tunnel: T5 {"GUI Ref"=refnum, "Status"=0, "Head Ref"=refnum, "Slider Ref"=refnum} ("Cluster") -> [w291]
    tunnel: w108 -> [w289] mode=indexing
    tunnel: [w290] -> w3 mode=indexing
    tunnel: w91 -> [w288] mode=indexing
    tunnel: w79 -> [w287] mode=indexing
    n230 = Bundle By Name(cluster=w291, "GUI Ref"=w289, "Head Ref"=w288, "Slider Ref"=w287) -> (w290:T5)
  }
  n231 = Bundle By Name(cluster=T4 {"Laser"=refnum, "PreAmp"=refnum, "MainAmp"=refnum, "Emergency Off"=refnum, "Exp 1"=refnum, "Exp 2"=refnum, "Exp 3"=refnum, "Exp 4"=refnum, "Timing Mode GUI Ref"=refnum} ("GUI Refs"), "Emergency Off"=w55, "Laser"=w54, "PreAmp"=w53, "MainAmp"=w52, "Exp 1"=w51, "Exp 2"=w50, "Exp 3"=w49, "Exp 4"=w48) -> (w27:T4)
  n232 = control-ref of="Mercury"() -> (w24:refnum<vi>)
  n233 = call "PH_Class.Register Event.vi"("i ref in"="object ref", "error in (no error)"="error in (no error)") -> ("i ref out"=w30:refnum<vi>, "Event Registration Refnum"=w29:refnum<event-registration>, "error out"=w31:errorcluster)  [unwired: 15 in]
  n234 = while {
    tunnel: w30 -> [w320]
    tunnel: [w319] -> w61
    tunnel: w31 -> [w322]
    tunnel: [w321] -> w258
    tunnel: w29 -> [w318]
    tunnel: [w317] -> w28
    tunnel: w27 -> [w316]
    tunnel: w24 -> [w315]
    tunnel: w23 -> [w314]
    tunnel: w22 -> [w313]
    tunnel: w21 -> [w312]
    tunnel: w20 -> [w311]
    tunnel: w19 -> [w310]
    tunnel: w18 -> [w309]
    tunnel: w17 -> [w308]
    tunnel: w16 -> [w307]
    tunnel: w15 -> [w306]
    tunnel: w14 -> [w305]
    tunnel: w13 -> [w304]
    tunnel: w12 -> [w303]
    tunnel: w11 -> [w302]
    tunnel: w10 -> [w301]
    tunnel: w9 -> [w300]
    tunnel: w8 -> [w299]
    tunnel: w7 -> [w298]
    tunnel: w6 -> [w297]
    tunnel: w5 -> [w296]
    tunnel: w4 -> [w295]
    tunnel: w3 -> [w294]
    tunnel: w2 -> [w293]
    tunnel: w1 -> [w292]
    stop <- w323 stop-if-true
    n235 = event shown="[4] \"PILo_enable_exp1\", \"PILo_enable_exp2\", \"PILo_enable_exp3\", \"PILo_enable_exp4\": Value Change" {
      selector: w318 -> [_ _ _ _ _ _ _ _ _ _ _ _]
      dyn-events: [_ _ _ _ _ _ _ _ _ _ _ _] -> w317
      timeout: _ -> [_ _ _ _ _ _ _ _ _ _ _ _]
      tunnel: ["Delete" _ _ _ _ _ _ _ _ _ _ _] -> w323
      tunnel: w320 -> [w327 w341 w352 w396 w442 w490 w493 w508 w523 w541 w577 w636]
      tunnel: w322 -> [w326 w340 w351 w395 w441 w489 w492 w507 w522 w540 w576 w635]
      tunnel: [w325 w337 w348 w392 w438 w486 w495 w510 w525 w543 w579 w607] -> w321
      tunnel: [w324 w338 w349 w393 w439 w487 w496 w511 w526 w544 w580 w605] -> w319
      tunnel: w316 -> [_ _ _ _ _ _ _ _ _ _ _ w632]
      tunnel: w315 -> [_ _ _ _ _ _ _ _ _ _ _ w631]
      tunnel: w314 -> [_ _ _ _ _ _ _ _ _ _ _ w630]
      tunnel: w313 -> [_ _ _ _ _ _ _ _ _ _ _ w629]
      tunnel: w312 -> [_ _ _ _ _ _ _ _ _ _ _ w628]
      tunnel: w311 -> [_ _ _ _ _ _ _ _ _ _ _ w627]
      tunnel: w310 -> [_ _ _ _ _ _ _ _ _ _ _ w626]
      tunnel: w309 -> [_ _ _ _ _ _ _ _ _ _ _ w625]
      tunnel: w308 -> [_ _ _ _ _ _ _ _ _ _ _ w624]
      tunnel: w307 -> [_ _ _ _ _ _ _ _ _ _ _ w623]
      tunnel: w306 -> [_ _ _ _ _ _ _ _ _ _ _ w622]
      tunnel: w305 -> [_ _ _ _ _ _ _ _ _ _ _ w621]
      tunnel: w304 -> [_ _ _ _ _ _ _ _ _ _ _ w620]
      tunnel: w303 -> [_ _ _ _ _ _ _ _ _ _ _ w619]
      tunnel: w302 -> [_ _ _ _ _ _ _ _ _ _ _ w618]
      tunnel: w301 -> [_ _ _ _ _ _ _ _ _ _ _ w617]
      tunnel: w300 -> [_ _ _ _ _ _ _ _ _ _ _ w616]
      tunnel: w299 -> [_ _ _ _ _ _ _ _ _ _ _ w615]
      tunnel: w298 -> [_ _ _ _ _ _ _ _ _ _ _ w614]
      tunnel: w297 -> [_ _ _ _ _ _ _ _ _ _ _ w613]
      tunnel: w296 -> [_ _ _ _ _ _ _ _ _ _ _ w612]
      tunnel: w295 -> [_ _ _ _ _ _ _ _ _ _ _ w611]
      tunnel: w294 -> [_ _ _ _ _ _ _ _ _ _ _ w610]
      tunnel: w293 -> [_ _ _ _ _ _ _ _ _ _ _ w609]
      tunnel: w292 -> [_ _ _ _ _ _ _ _ _ _ _ w608]
      event "Delete": Value Change {
        n236 = event-data() -> ()  [unwired: 1 in, 1 out]
        n237 = call "PH_Class.Delete GUI.vi"("VI in"=w327, "error in (no error)"=w326) -> ("VI out"=w324:refnum<vi>, "error out"=w325:errorcluster)  [unwired: 16 in]
      }
      event "PILo_enable_AllLaser": Value Change {
        n238 = event-data() -> ("CtlRef"=w335:refnum<vi>, "OldVal"=w331:bool, "NewVal"=w336:bool)  [unwired: 1 in]
        n239 = call "PH_PILS.get i attribute.vi"("i ref in"=w341, "error in (no error)"=w340) -> ("i ref out"=w339:refnum<vi>, "i attribute"=w330:T6, "error out"=w334:errorcluster)  [unwired: 15 in]
        n240 = Unbundle By Name(w330) -> ("Beckhoff-Instance Internal"=w329:string)
        n241 = property class="Bool (strict)"(reference=w335, error in=w334, "Value"=w331) -> (error out=w333:errorcluster, "Label.Text"=w332:string)  [unwired: 1 out]
        n242 = call "PH_Beckhoff.evt Call Set Boolean Value.vi"("i ref in"=w339, "Beckhoff Instance"=w329, "Tagname to set"=w332, "Value"=w336, "error in"=w333) -> ("i ref out"=w338:refnum<vi>, "error out"=w337:errorcluster)  [unwired: 13 in]
      }
      event "PILo_enable_Preamp": Value Change {
        n243 = event-data() -> ("CtlRef"=w344:refnum<vi>, "OldVal"=w345:bool, "NewVal"=w347:bool)  [unwired: 1 in]
        n244 = call "PH_PILS.get i attribute.vi"("i ref in"=w352, "error in (no error)"=w351) -> ("i ref out"=w350:refnum<vi>, "i attribute"=w343:T6, "error out"=w346:errorcluster)  [unwired: 15 in]
        n245 = Unbundle By Name(w343) -> ("Beckhoff-Instance Internal"=w342:string)
        n246 = case shown="False" w347 {
          selector: w347 -> [w359 w374]
          tunnel: w350 -> [w362 w373]
          tunnel: [w361 w376] -> w349
          tunnel: [w360 w375] -> w348
          tunnel: w346 -> [w358 w369]
          tunnel: w342 -> [w353 w363]
          tunnel: w345 -> [w355 w365]
          tunnel: w344 -> [w356 w364]
          frame False {
            n247 = property class="Bool (strict)"(reference=w356, error in=w358, "Value"=w355) -> (error out=w357:errorcluster, "Label.Text"=w354:string)  [unwired: 1 out]
            n248 = call "PH_Beckhoff.evt Call Set Boolean Value.vi"("i ref in"=w362, "Beckhoff Instance"=w353, "Tagname to set"=w354, "Value"=w359, "error in"=w357) -> ("i ref out"=w361:refnum<vi>, "error out"=w360:errorcluster)  [unwired: 13 in]
          }
          frame True {
            w371 = u16 0 items=["PreAmp", "MainAmp", "ext Exp"] ("System to enable")
            n249 = call "PH_PILS.Enabling Checking.vi"("i ref in"=w373, "System to enable"=w371, "error in"=w369) -> ("i ref out"=w372:refnum<vi>, "Enabling allowed"=w370:bool, "error out"=w368:errorcluster)  [unwired: 14 in]
            n250 = property class="Bool (strict)"(reference=w364, error in=w368, "Value"=w365) -> (error out=w367:errorcluster, "Label.Text"=w366:string)  [unwired: 1 out]
            n251 = case shown="True" w370 {
              tunnel: [w378 w385] -> w376
              tunnel: [w377 w384] -> w375
              tunnel: w363 -> [_ w383]
              tunnel: w366 -> [_ w382]
              tunnel: w374 -> [_ w381]
              tunnel: w367 -> [w377 w380]
              tunnel: w372 -> [w378 w379]
              frame False {
              }
              frame True {
                n252 = call "PH_Beckhoff.evt Call Set Boolean Value.vi"("i ref in"=w379, "Beckhoff Instance"=w383, "Tagname to set"=w382, "Value"=w381, "error in"=w380) -> ("i ref out"=w385:refnum<vi>, "error out"=w384:errorcluster)  [unwired: 13 in]
              }
            }
          }
        }
      }
      event "PILo_enable_mainamp": Value Change {
        n253 = event-data() -> ("CtlRef"=w388:refnum<vi>, "OldVal"=w389:bool, "NewVal"=w391:bool)  [unwired: 1 in]
        n254 = call "PH_PILS.get i attribute.vi"("i ref in"=w396, "error in (no error)"=w395) -> ("i ref out"=w394:refnum<vi>, "i attribute"=w387:T6, "error out"=w390:errorcluster)  [unwired: 15 in]
        n255 = Unbundle By Name(w387) -> ("Beckhoff-Instance Internal"=w386:string)
        n256 = case shown="True" w391 {
          selector: w391 -> [w403 w418]
          tunnel: w394 -> [w406 w417]
          tunnel: [w405 w420] -> w393
          tunnel: [w404 w419] -> w392
          tunnel: w390 -> [w402 w413]
          tunnel: w386 -> [w397 w407]
          tunnel: w389 -> [w399 w409]
          tunnel: w388 -> [w400 w408]
          frame False {
            n257 = property class="Bool (strict)"(reference=w400, error in=w402, "Value"=w399) -> (error out=w401:errorcluster, "Label.Text"=w398:string)  [unwired: 1 out]
            n258 = call "PH_Beckhoff.evt Call Set Boolean Value.vi"("i ref in"=w406, "Beckhoff Instance"=w397, "Tagname to set"=w398, "Value"=w403, "error in"=w401) -> ("i ref out"=w405:refnum<vi>, "error out"=w404:errorcluster)  [unwired: 13 in]
          }
          frame True {
            w415 = u16 1 items=["PreAmp", "MainAmp", "ext Exp"] ("System to enable")
            n259 = call "PH_PILS.Enabling Checking.vi"("i ref in"=w417, "System to enable"=w415, "error in"=w413) -> ("i ref out"=w416:refnum<vi>, "Enabling allowed"=w414:bool, "error out"=w412:errorcluster)  [unwired: 14 in]
            n260 = property class="Bool (strict)"(reference=w408, error in=w412, "Value"=w409) -> (error out=w411:errorcluster, "Label.Text"=w410:string)  [unwired: 1 out]
            n261 = case shown="True" w414 {
              tunnel: [w422 w429] -> w420
              tunnel: [w421 w428] -> w419
              tunnel: w407 -> [_ w427]
              tunnel: w410 -> [_ w426]
              tunnel: w418 -> [_ w425]
              tunnel: w411 -> [w421 w424]
              tunnel: w416 -> [w422 w423]
              frame False {
              }
              frame True {
                n262 = call "PH_Beckhoff.evt Call Set Boolean Value.vi"("i ref in"=w423, "Beckhoff Instance"=w427, "Tagname to set"=w426, "Value"=w425, "error in"=w424) -> ("i ref out"=w429:refnum<vi>, "error out"=w428:errorcluster)  [unwired: 13 in]
              }
            }
          }
        }
      }
      event "PILo_enable_exp1", "PILo_enable_exp2", "PILo_enable_exp3", "PILo_enable_exp4": Value Change {
        n263 = event-data() -> ("CtlRef"=w434:refnum<vi>, "OldVal"=w435:bool, "NewVal"=w437:bool)  [unwired: 1 in]
        n264 = call "PH_PILS.get i attribute.vi"("i ref in"=w442, "error in (no error)"=w441) -> ("i ref out"=w440:refnum<vi>, "i attribute"=w433:T6, "error out"=w436:errorcluster)  [unwired: 15 in]
        n265 = Unbundle By Name(w433) -> ("Beckhoff-Instance Internal"=w431:string, "Beckhoff-Instance External"=w430:string)
        n266 = case shown="\"\", \"N/A\"" w430 {
          selector: w430 -> [w443 _]
          tunnel: [w443 w444] -> w432
          tunnel: w431 -> [_ w444]
          frame Default {
          }
          frame "", "N/A" {
          }
        }
        n267 = case shown="True" w437 {
          selector: w437 -> [w451 w466]
          tunnel: w440 -> [w454 w465]
          tunnel: [w453 w468] -> w439
          tunnel: [w452 w467] -> w438
          tunnel: w436 -> [w450 w461]
          tunnel: w432 -> [w445 w455]
          tunnel: w435 -> [w447 w457]
          tunnel: w434 -> [w448 w456]
          frame False {
            n268 = property class="Bool (strict)"(reference=w448, error in=w450, "Value"=w447) -> (error out=w449:errorcluster, "Label.Text"=w446:string)  [unwired: 1 out]
            n269 = call "PH_Beckhoff.evt Call Set Boolean Value.vi"("i ref in"=w454, "Beckhoff Instance"=w445, "Tagname to set"=w446, "Value"=w451, "error in"=w449) -> ("i ref out"=w453:refnum<vi>, "error out"=w452:errorcluster)  [unwired: 13 in]
          }
          frame True {
            w463 = u16 2 items=["PreAmp", "MainAmp", "ext Exp"] ("System to enable")
            n270 = call "PH_PILS.Enabling Checking.vi"("i ref in"=w465, "System to enable"=w463, "error in"=w461) -> ("i ref out"=w464:refnum<vi>, "Enabling allowed"=w462:bool, "error out"=w460:errorcluster)  [unwired: 14 in]
            n271 = property class="Bool (strict)"(reference=w456, error in=w460, "Value"=w457) -> (error out=w459:errorcluster, "Label.Text"=w458:string)  [unwired: 1 out]
            n272 = case shown="True" w462 {
              tunnel: [w470 w477] -> w468
              tunnel: [w469 w476] -> w467
              tunnel: w455 -> [_ w475]
              tunnel: w458 -> [_ w474]
              tunnel: w466 -> [_ w473]
              tunnel: w459 -> [w469 w472]
              tunnel: w464 -> [w470 w471]
              frame False {
              }
              frame True {
                n273 = call "PH_Beckhoff.evt Call Set Boolean Value.vi"("i ref in"=w471, "Beckhoff Instance"=w475, "Tagname to set"=w474, "Value"=w473, "error in"=w472) -> ("i ref out"=w477:refnum<vi>, "error out"=w476:errorcluster)  [unwired: 13 in]
              }
            }
          }
        }
      }
      event "PILo_enable_MainEmergency": Value Change {
        n274 = event-data() -> ("CtlRef"=w482:refnum<vi>, "OldVal"=w483:bool, "NewVal"=w485:bool)  [unwired: 1 in]
        n275 = call "PH_PILS.get i attribute.vi"("i ref in"=w490, "error in (no error)"=w489) -> ("i ref out"=w488:refnum<vi>, "i attribute"=w479:T6, "error out"=w484:errorcluster)  [unwired: 15 in]
        n276 = Unbundle By Name(w479) -> ("Beckhoff-Instance Internal"=w478:string)
        n277 = property class="Bool (strict)"(reference=w482, error in=w484, "Value"=w483) -> (error out=w481:errorcluster, "Label.Text"=w480:string)  [unwired: 1 out]
        n278 = call "PH_Beckhoff.evt Call Set Boolean Value.vi"("i ref in"=w488, "Beckhoff Instance"=w478, "Tagname to set"=w480, "Value"=w485, "error in"=w481) -> ("i ref out"=w487:refnum<vi>, "error out"=w486:errorcluster)  [unwired: 13 in]
      }
      event "PILo_activate_laser_power": Value Change {
        n279 = event-data() -> ("CtlRef"=w494:refnum<vi>)  [unwired: 1 in]
        n280 = case shown="True" "PILo_activate_laser_power" {
          tunnel: [w498 w505] -> w496
          tunnel: [w497 w504] -> w495
          tunnel: w494 -> [_ w502]
          tunnel: w493 -> [w498 w500]
          tunnel: w492 -> [w497 w499]
          frame False {
          }
          frame True {
            n281 = property class="Bool"(reference=w502, error in=w499) -> (error out=w503:errorcluster, "Label.Text"=w501:string)  [unwired: 1 out]
            n282 = call "PH_PILS.Activate Tag.vi"("i ref in"=w500, "Tag Name"=w501, "error in (no error)"=w503) -> ("i ref out"=w505:refnum<vi>, "error out"=w504:errorcluster)  [unwired: 15 in]
          }
        }
      }
      event "PILo_activate_extEmergencies": Value Change {
        n283 = event-data() -> ("CtlRef"=w509:refnum<vi>)  [unwired: 1 in]
        n284 = case shown="True" "PILo_activate_extEmergencies" {
          tunnel: [w513 w520] -> w511
          tunnel: [w512 w519] -> w510
          tunnel: w509 -> [_ w518]
          tunnel: w508 -> [w513 w515]
          tunnel: w507 -> [w512 w516]
          frame False {
          }
          frame True {
            n285 = property class="Bool"(reference=w518, error in=w516) -> (error out=w514:errorcluster, "Label.Text"=w517:string)  [unwired: 1 out]
            n286 = call "PH_PILS.Activate Tag.vi"("i ref in"=w515, "Tag Name"=w517, "error in (no error)"=w514) -> ("i ref out"=w520:refnum<vi>, "error out"=w519:errorcluster)  [unwired: 15 in]
          }
        }
      }
      event "PILo_unlock_HVDoor": Value Change {
        n287 = event-data() -> ("CtlRef"=w524:refnum<vi>)  [unwired: 1 in]
        n288 = case shown="True" "PILo_unlock_HVDoor" {
          tunnel: [w528 w535] -> w526
          tunnel: [w527 w534] -> w525
          tunnel: w524 -> [_ w533]
          tunnel: w523 -> [w528 w531]
          tunnel: w522 -> [w527 w530]
          frame False {
          }
          frame True {
            n289 = property class="Bool"(reference=w533, error in=w530) -> (error out=w529:errorcluster, "Label.Text"=w532:string)  [unwired: 1 out]
            n290 = call "PH_PILS.Activate Tag.vi"("i ref in"=w531, "Tag Name"=w532, "error in (no error)"=w529) -> ("i ref out"=w535:refnum<vi>, "error out"=w534:errorcluster)  [unwired: 15 in]
          }
        }
      }
      event "PILo_lock_HVDoor": Value Change {
        n291 = event-data() -> ("CtlRef"=w542:refnum<vi>)  [unwired: 1 in]
        n292 = property class="Bool"(reference=w542, error in=w540) -> (error out=w539:errorcluster, "Label.Text"=w536:string)  [unwired: 1 out]
        n293 = case shown="True" "PILo_lock_HVDoor" {
          tunnel: [w546 w556] -> w544
          tunnel: [w545 w555] -> w543
          tunnel: w541 -> [w546 w548]
          tunnel: w539 -> [w545 w547]
          tunnel: "PILo_activate_AllDoors" -> [_ w554]
          tunnel: w536 -> [_ w549]
          frame False {
          }
          frame True {
            n294 = flat-sequence {
              tunnel: w548 -> [w559]
              tunnel: w547 -> [w558]
              tunnel: w554 -> [w557]
              tunnel: [w561] -> w553
              tunnel: [w560] -> w552
              tunnel: w553 -> [w564]
              tunnel: w552 -> [w563]
              tunnel: [w564] -> w551
              tunnel: [w563] -> w550
              tunnel: [w566] -> w555
              tunnel: [w567] -> w556
              tunnel: w551 -> [w569]
              tunnel: w550 -> [w568]
              tunnel: w549 -> [w565]
              frame #0 {
                n295 = call "PH_PILS.Activate Tag.vi"("i ref in"=w559, "Tag Name"=w557, "error in (no error)"=w558) -> ("i ref out"=w561:refnum<vi>, "error out"=w560:errorcluster)  [unwired: 15 in]
              }
              frame #1 {
                n296 = Wait (ms)(milliseconds to wait=u32 250) -> ()  [unwired: 1 out]
              }
              frame #2 {
                n297 = call "PH_PILS.Activate Tag.vi"("i ref in"=w569, "Tag Name"=w565, "error in (no error)"=w568) -> ("i ref out"=w567:refnum<vi>, "error out"=w566:errorcluster)  [unwired: 15 in]
              }
            }
          }
        }
      }
      event "PILo_activate_MainEmergency": Value Change {
        n298 = event-data() -> ("CtlRef"=w578:refnum<vi>)  [unwired: 1 in]
        n299 = property class="Bool"(reference=w578, error in=w576) -> (error out=w575:errorcluster, "Label.Text"=w573:string)  [unwired: 1 out]
        n300 = Build Array("PILo_activate_subEmergencies", "PILo_activate_extEmergencies", w573) -> (w572:string[])
        n301 = case shown="True" "PILo_activate_MainEmergency" {
          tunnel: [w582 w592] -> w580
          tunnel: [w581 w591] -> w579
          tunnel: w577 -> [w582 w596]
          tunnel: w575 -> [w581 w599]
          tunnel: w572 -> [_ w598]
          frame False {
          }
          frame True {
            n302 = call "PH_PILS.get i attribute.vi"("i ref in"=w596, "error in (no error)"=w599) -> ("i ref out"=w595:refnum<vi>, "i attribute"=w584:T6, "error out"=w597:errorcluster)  [unwired: 15 in]
            n303 = Unbundle By Name(w584) -> ("Logfile"=w583:path)
            n304 = Open/Create/Replace File(file path (use dialog)=w583) -> (refnum out=w588:refnum<file>, error out=w587:errorcluster)  [unwired: 5 in, 1 out]
            n305 = Set File Position(refnum=w588, from (0:start)=enum16{"start", "end", "current"}."end", error in=w587) -> (refnum out=w586:refnum<file>, error out=w585:errorcluster)  [unwired: 1 in]
            n306 = call "PH_PILS.Dialog EO.vi"() -> ("EO Comment"=w589:string)
            n307 = for {
              tunnel: w598 -> [w600] mode=indexing
              shift-right: [w604] -> w592
              shift-left: w595 -> [w602]
              shift-right: [w603] -> w591
              shift-left: w597 -> [w601]
              n308 = call "PH_PILS.Activate Tag.vi"("i ref in"=w602, "Tag Name"=w600, "error in (no error)"=w601) -> ("i ref out"=w604:refnum<vi>, "error out"=w603:errorcluster)  [unwired: 15 in]
            }
            n309 = Write to Text File(file (use dialog)=w586, text=w589, error in=w585) -> (refnum out=w594:refnum<file>, error out=w593:errorcluster)  [unwired: 1 in, 1 out]
            n310 = Close File(refnum=w594, error in=w593) -> ()  [unwired: 2 out]
          }
        }
      }
      event User Event {
        n311 = event-data() -> ("Class"=w634:string)  [unwired: 1 in]
        n312 = case shown="\"PH_PILS\"" w634 {
          selector: w634 -> [w637 _]
          tunnel: w636 -> [w642 w670]
          tunnel: [w641 w644] -> w606
          tunnel: w635 -> [w640 w669]
          tunnel: [w639 w643] -> w633
          tunnel: w632 -> [w638 _]
          tunnel: w631 -> [_ w668]
          tunnel: w630 -> [_ w667]
          tunnel: w629 -> [_ w666]
          tunnel: w628 -> [_ w665]
          tunnel: w627 -> [_ w664]
          tunnel: w626 -> [_ w663]
          tunnel: w625 -> [_ w662]
          tunnel: w624 -> [_ w661]
          tunnel: w623 -> [_ w660]
          tunnel: w622 -> [_ w659]
          tunnel: w621 -> [_ w658]
          tunnel: w620 -> [_ w657]
          tunnel: w619 -> [_ w656]
          tunnel: w618 -> [_ w655]
          tunnel: w617 -> [_ w654]
          tunnel: w616 -> [_ w653]
          tunnel: w615 -> [_ w652]
          tunnel: w614 -> [_ w651]
          tunnel: w613 -> [_ w650]
          tunnel: w612 -> [_ w649]
          tunnel: w611 -> [_ w648]
          tunnel: w610 -> [_ w647]
          tunnel: w609 -> [_ w646]
          tunnel: w608 -> [_ w645]
          frame Default {
            n313 = call "PH_SystemInformation.set GUI Refs.vi"("i ref in"=w642, "Class"=w637, "System Information GUI Refs"=w638, "error in (no error)"=w640) -> ("i ref out"=w641:refnum<vi>, "error out"=w639:errorcluster)  [unwired: 14 in]
          }
          frame "PH_PILS" {
            n314 = call "PH_PILS.get data to modify.vi"("i ref in"=w670, "ms timeout (10000)"=-1, "error in (no error)"=w669) -> ("i ref out"=w675:refnum<vi>, "i attribute"=w672:T6, "error out"=w674:errorcluster)  [unwired: 13 in, 1 out]
            n315 = Bundle By Name(cluster=w672, "Mercury"=w668, "EO-Likes"=w667, "Boolean"=w666, "GUI Refs Exp. Shutters.1"=w665, "GUI Refs Exp. Shutters.2"=w664, "GUI Refs Exp. Shutters.3"=w663, "GUI Refs Exp. Shutters.4"=w662, "Tristate2Run GUI Refs"=w661, "TristateNormal"=w660, "Operation Mode.GUI.Ref State"=w659, "Operation Mode.GUI.Ref"=w658, "Submode.GUI.Ref State"=w657, "Submode.GUI.Ref"=w656, "Experiment.GUI.Ref State"=w655, "Experiment.GUI.Ref"=w654, "Door Tags"=w653, "Beamline GUI Refs"=w652, "Special Boolean"=w651, "Laserpower"=w650, "Shutter"=w649, "Tristate EO Like"=w648, "PP"=w647, "Switch Knobs"=w646, "Latch Knob GUI Refs"=w645) -> (w671:T6)
            n316 = call "PH_PILS.set modified data.vi"("i ref in"=w675, "i attribute"=w671, "error in (no error)"=w674) -> ("i ref out"=w644:refnum<vi>, "error out"=w643:errorcluster)  [unwired: 15 in]
          }
        }
        n317 = call "PH_Class.set GUI Refs stored Occurence.vi"("i ref in"=w606, "error in (no error)"=w633) -> ("i ref out"=w605:refnum<vi>, "error out"=w607:errorcluster)  [unwired: 16 in]
      }
    }
  }
  "error out" <- w258
  n318 = property on="PIL_Exp1_DoorOpen" class="ColBox"("Disabled"=w77) -> ()  [unwired: 2 in, 2 out]
  n319 = property on="PIL_Exp2_DoorOpen" class="ColBox"("Disabled"=w77) -> ()  [unwired: 2 in, 2 out]
  n320 = property on="PIL_Exp3_DoorOpen" class="ColBox"("Disabled"=w77) -> ()  [unwired: 2 in, 2 out]
  n321 = property on="PP_PA-45mm-PILC_DumpRoss_DE_closed" class="ColBox"("Visible"=w98) -> ()  [unwired: 2 in, 2 out]
  n322 = property on="PPMA_Rods_b_down" class="ColBox"("Visible"=w98) -> ()  [unwired: 2 in, 2 out]
  n323 = property on="Beamline Einschuss Exp. 1" class="ColBox"("Visible"=w171) -> ()  [unwired: 2 in, 2 out]
  n324 = property on="Beamline Einschuss Exp. 2" class="ColBox"("Visible"=w171) -> ()  [unwired: 2 in, 2 out]
  n325 = property on="Beamline Einschuss Exp. 3" class="ColBox"("Visible"=w171) -> ()  [unwired: 2 in, 2 out]
  n326 = property on="Beamline Exp. 1" class="ColBox"("Visible"=w171) -> ()  [unwired: 2 in, 2 out]
  n327 = property on="Beamline Exp. 2" class="ColBox"("Visible"=w171) -> ()  [unwired: 2 in, 2 out]
  n328 = property on="Beamline Exp. 3" class="ColBox"("Visible"=w171) -> ()  [unwired: 2 in, 2 out]
  n329 = control-ref of="PPMA_PU7_PSU_HV_on"() -> (w45:refnum<vi>)
  n330 = control-ref of="PPMA_PU8_PSU_HV_on"() -> (w44:refnum<vi>)
  n331 = control-ref of="PPMA_PU9_PSU_HV_on"() -> (w43:refnum<vi>)
  n332 = control-ref of="PPMA_PU10_PSU_HV_on"() -> (w42:refnum<vi>)
  n333 = control-ref of="PPMA_PU7_PSU_HV_on Head"() -> (w40:refnum<vi>)
  n334 = control-ref of="PPMA_PU8_PSU_HV_on Head"() -> (w39:refnum<vi>)
  n335 = control-ref of="PPMA_PU9_PSU_HV_on Head"() -> (w38:refnum<vi>)
  n336 = control-ref of="PPMA_PU10_PSU_HV_on Head"() -> (w37:refnum<vi>)
  n337 = control-ref of="PPMA_Rack4_DC_ok"() -> (w36:refnum<vi>)
  n338 = control-ref of="PPMA_Rack5_DC_ok"() -> (w35:refnum<vi>)
  n339 = Build Array(w45, w44, w43, w42, w40, w39, w38, w37, w36, w35) -> (w41:refnum<vi>[])
  n340 = for {
    tunnel: w41 -> [w677] mode=indexing
    n341 = property class="ColBox"(reference=w677, "Visible"=FALSE) -> ()  [unwired: 1 in, 2 out]
  }
  n342 = Unregister For Events(event registration refnum=w28) -> ()  [unwired: 1 in, 1 out]
  n343 = call "PH_Interaction.Super Destroy Me.vi"("i ref out"=w61) -> ()
